vi "Init Actor Core.vi"(8 "error in (no error)":errorcluster, 11 "Measure Object in":refnum<class "TestLabActor.lvclass">) -> (0 "error out":errorcluster, 3 "Measure Object out":refnum<class "TestLabActor.lvclass">)   [LabVIEW 2019]
uses:
  TestLabActor.lvclass
  Template Module/Template Module.lvclass
  C:/GitHub/LabActor/Template Module/Template Module.lvclass
  C:/Program Files/National Instruments/LabVIEW 2019/vi.lib/ActorFramework/Actor/Actor.lvclass
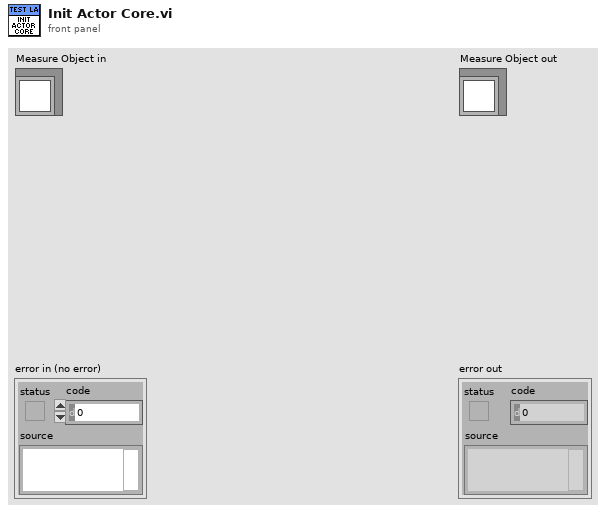
[diagram p1: front panel]
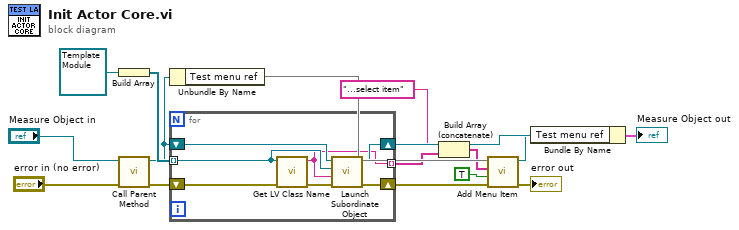
[diagram p0: block diagram]
diagram:
  n1 = Build Array(refnum<class "Template Module.lvclass"> refnum ("Template Module.lvclass")) -> (w12:refnum<class "Template Module.lvclass">[])
  n2 = call-parent "Call Parent Method"("error in (no error)"="error in (no error)", "Measure Object in"="Measure Object in") -> ("error out"=w14:errorcluster, "Measure Object out"=w11:refnum<class "TestLabActor.lvclass">)  [unwired: 8 in]
  n3 = Unbundle By Name(w11) -> ("Test menu ref"=w10)
  n4 = for {
    shift-right: [w23] -> w9
    shift-left: w14 -> [w19]
    shift-right: [w21] -> w8
    shift-left: w11 -> [w22]
    tunnel: w12 -> [w20] mode=indexing
    tunnel: [w17] -> w1 mode=indexing
    n5 = call <vilib>:"Get LV Class Name.vi"("error in (no error)"=w19, "object"=w20) -> ("error out"=w18:errorcluster, "class name"=w17:string)  [unwired: 8 in]
    n6 = call-dynamic "Launch Subordinate Object.vi"("error in (no error)"=w18, "Name"=w17, "Subordinate Object"=w20, "Template Module in"=w22) -> ("error out"=w23:errorcluster, "Template Module out"=w21:refnum<class "TestLabActor.lvclass">)  [unwired: 5 in, 1 out]
  }
  n7 = Build Array (concatenate)("...select item", w1) -> (w3:string[])
  n8 = call "Add Menu Item.vi"("error in (no error)"=w9, "Reset"=TRUE, "Item Names"=w3, "Queed Listbox ref"=w10) -> ("error out"=→"error out":errorcluster, "Queed Listbox ref out"=w7:refnum<vi>)  [unwired: 5 in, 1 out]
  n9 = Bundle By Name(cluster=w8, "Test menu ref"=w7) -> (→"Measure Object out":cluster{})
